vi "Set LED State.vi"(8 "error in (no error)":errorcluster, 10 "Get/Set":T2, 11 "Blink?":bool) -> (0 "error out":errorcluster, 3 "LED State Out":T1)   [LabVIEW 2016]
uses:
  Type Defs/State Action.ctl
  Valew Common/type defs/LED Status OOB.ctl
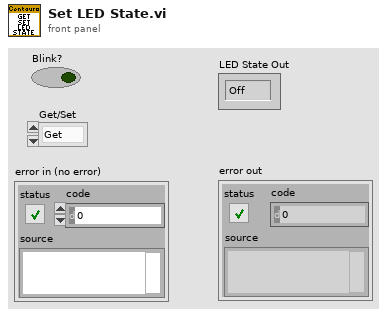
[diagram p1: front panel]
types:
  T1 = typedef "LED Status OOB.ctl" = enum32{"Off", "On", "Blink"}
  T2 = typedef "State Action.ctl" = enum16{"Get", "Set"}
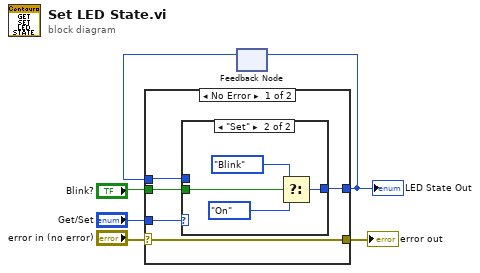
[diagram p0: block diagram]
diagram:
  n1 = feedback #1() -> (w5:T1)  [unwired: 1 in]
  n2 = case shown="No Error" "error in (no error)" {
    selector: "error in (no error)" -> [w9 w18]
    tunnel: [w11 w17] -> w6
    tunnel: w5 -> [w10 w17]
    tunnel: [w9 w18] -> w3
    tunnel: "Blink?" -> [w8 _]
    tunnel: "Get/Set" -> [w7 _]
    frame No Error {
      n3 = case shown="\"Set\"" w7 {
        tunnel: [w12 w14] -> w11
        tunnel: w8 -> [_ w13]
        tunnel: w10 -> [w12 _]
        frame "Get", Default {
        }
        frame "Set" {
          n4 = Select(t=LED_Status_OOB."Blink" ("Deep Rinse"), s=w13, f=LED_Status_OOB."On" ("Deep Rinse")) -> (s? t:f=w14:T1)
        }
      }
    }
    frame Error {
    }
  }
  "LED State Out" <- w6
  "error out" <- w3
  n5 = feedback-in #1(w6) -> ()
